vi "FRCts20_Backend_KeyGen.vi"(19 "Init?":bool) -> (26 "Keygen":string)   [LabVIEW 2013, in "FRCts20_Backend_Engine.lvlib"]
doc: "Generates a unique key for each call by incrementing a fgv counter by one."
uses:
  FRCts20_Backend_Engine.lvlib
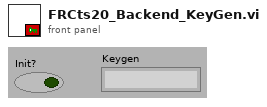
[diagram p1: front panel]
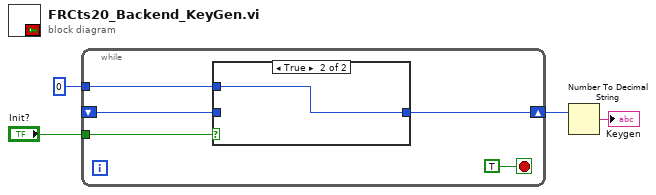
[diagram p0: block diagram]
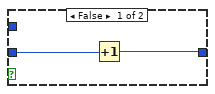
[diagram p2: hidden frame]
diagram:
  n1 = while {
    shift-right: [w6] -> w2
    shift-left: _ -> [w5]
    tunnel: u64 0 -> [w7]
    tunnel: "Init?" -> [w8]
    stop <- TRUE stop-if-true
    n2 = case shown="True" w8 {
      tunnel: w7 -> [_ w12]
      tunnel: [w10 w12] -> w6
      tunnel: w5 -> [w11 _]
      frame False {
        n3 = Increment(x=w11) -> (x+1=w10:u64)
      }
      frame True {
      }
    }
  }
  n4 = Number To Decimal String(number=w2) -> (decimal integer string=→"Keygen":string)  [unwired: 1 in]
